vi "Start load.vi"(8 "error in (no error)":errorcluster) -> (0 "error out":errorcluster)   [LabVIEW 2019]
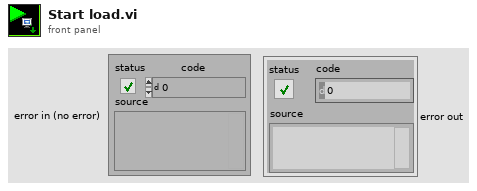
[diagram p1: front panel]
types:
  T1 = enum32{"Invalid", "Standard", "Closed", "Hidden", "Minimized", "Maximized"}
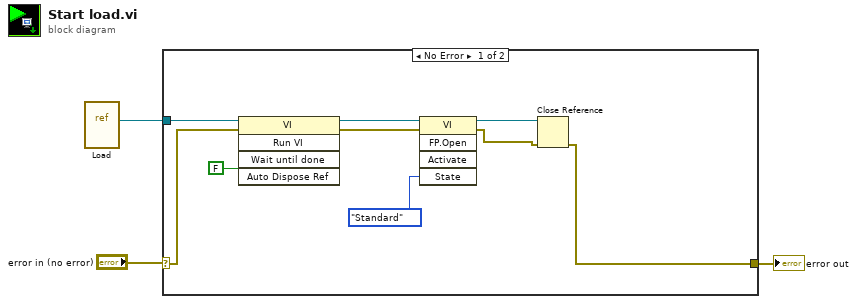
[diagram p0: block diagram]
diagram:
  n1 = vi-ref "Load.vi"() -> (w1:refnum<vi>)
  n2 = case shown="No Error" "error in (no error)" {
    selector: "error in (no error)" -> [w4 w13]
    tunnel: w1 -> [w12 _]
    tunnel: [w5 w13] -> w2
    frame No Error {
      n3 = invoke class="VI" method="Run VI"(reference=w12, error in=w4, "Wait until done"=FALSE ("Wait Until Done")) -> (reference out=w10:refnum<vi>, error out=w9:errorcluster)  [unwired: 2 in, 3 out]
      n4 = invoke class="VI" method="FP.Open"(reference=w10, error in=w9, "State"=T1."Standard") -> (reference out=w7:refnum<vi>, error out=w6:errorcluster)  [unwired: 2 in, 3 out]
      n5 = Close Reference(reference=w7, error in (no error)=w6) -> (error out=w5:errorcluster)
    }
    frame Error {
    }
  }
  "error out" <- w2
